vi "SaveTemplate.vi"(11 "Template Name":string) -> ()   [LabVIEW 2019]
uses:
  <userlib>/MicroPython/VIs/ColorText/Code.xctl
panel:
  in  "VISA resource name":refnum<visa-resource-name>
  in  "Open":bool
  in  "Save Button":bool
  in  "Code":string(xcontrol)
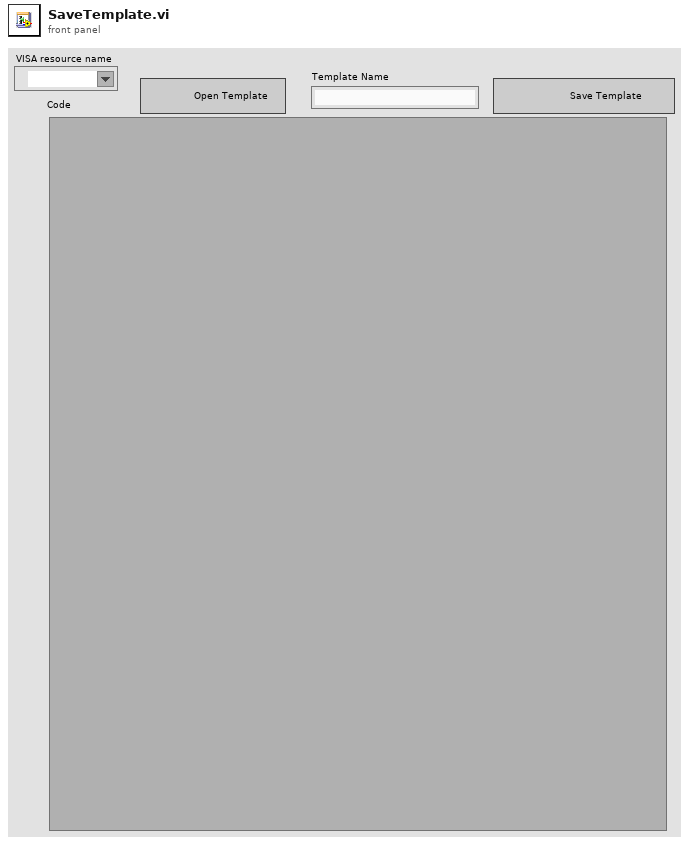
[diagram p1: front panel]
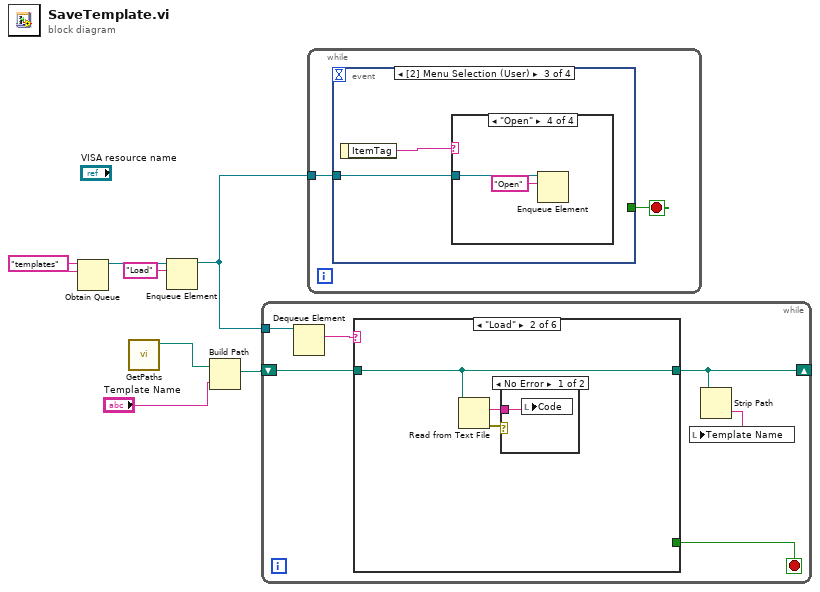
[diagram p0: block diagram]
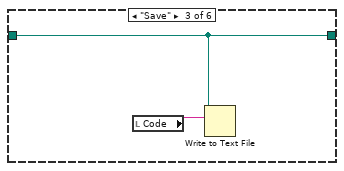
[diagram p4: hidden frame]
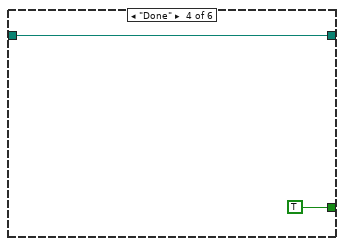
[diagram p5: hidden frame]
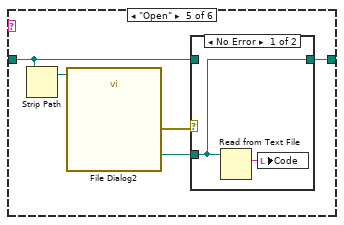
[diagram p6: hidden frame]
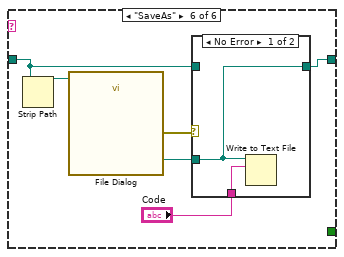
[diagram p8: hidden frame]
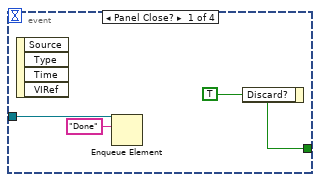
[diagram p10: hidden frame]
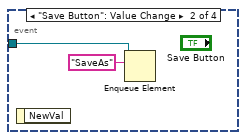
[diagram p11: hidden frame]
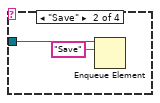
[diagram p13: hidden frame]
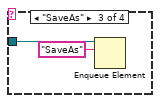
[diagram p14: hidden frame]
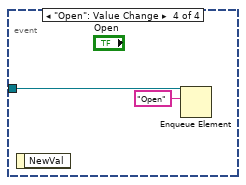
[diagram p15: hidden frame]
diagram:
  w2 = "templates" ("name (unnamed)")
  n1 = Obtain Queue(name (unnamed)=w2, element data type=w2) -> (queue out=w3:refnum<queue>)  [unwired: 3 in, 2 out]
  n2 = call <userlib>:"GetPaths.vi"() -> ("Templates path"=w7:path)  [unwired: 10 in, 1 out]
  n3 = Enqueue Element(queue=w3, element="Load") -> (queue out=w1:refnum<queue>)  [unwired: 2 in, 2 out]
  n4 = Build Path(base path=w7, name or relative path="Template Name") -> (appended path=w5:path)
  n5 = while {
    shift-right: [w9] -> _
    shift-left: w5 -> [w12]
    tunnel: w1 -> [w10]
    stop <- w8 stop-if-true
    n6 = Dequeue Element(queue=w10) -> (element=w13:string)  [unwired: 2 in, 3 out]
    n7 = case shown="\"Load\"" w13 {
      tunnel: [w14 w15 w19 w22 w23 w32] -> w9
      tunnel: w12 -> [w14 w15 w19 w22 w24 w31]
      tunnel: [_ _ _ TRUE _ _] -> w8
      frame Default {
      }
      frame "Load" {
        n8 = Read from Text File(file (use dialog)=w15) -> (text=w16:string, error out=w17:errorcluster)  [unwired: 3 in, 2 out]
        n9 = case shown="No Error" w17 {
          tunnel: w16 -> [w18 _]
          frame No Error {
            n10 = local write "Code"(w18) -> ()
          }
          frame Error {
          }
        }
      }
      frame "Save" {
        n11 = local read "Code"() -> (w20:string)
        n12 = Write to Text File(file (use dialog)=w19, text=w20) -> ()  [unwired: 2 in, 3 out]
      }
      frame "Done" {
      }
      frame "Open" {
        n13 = Strip Path(path=w24) -> (stripped path=w26:path)  [unwired: 1 out]
        n14 = call "File Dialog2"("start path"=w26) -> ("selected path"=w25:path, "error out"=w27:errorcluster)  [unwired: 11 in, 2 out]
        n15 = case shown="No Error" w27 {
          tunnel: w25 -> [w28 _]
          tunnel: [w28 w30] -> w23
          tunnel: w24 -> [_ w30]
          frame No Error {
            n16 = Read from Text File(file (use dialog)=w28) -> (text=w29:string)  [unwired: 3 in, 3 out]
            n17 = local write "Code"(w29) -> ()
          }
          frame Error {
          }
        }
      }
      frame "SaveAs" {
        n18 = Strip Path(path=w31) -> (stripped path=w35:path)  [unwired: 1 out]
        n19 = call "File Dialog"("start path"=w35) -> ("selected path"=w33:path, "error out"=w36:errorcluster)  [unwired: 11 in, 2 out]
        n20 = case shown="No Error" w36 {
          tunnel: w33 -> [w37 _]
          tunnel: "Code" -> [w38 _]
          tunnel: [w37 w39] -> w32
          tunnel: w31 -> [_ w39]
          frame No Error {
            n21 = Write to Text File(file (use dialog)=w37, text=w38) -> ()  [unwired: 2 in, 3 out]
          }
          frame Error {
          }
        }
      }
    }
    n22 = Strip Path(path=w9) -> (name=w11:string)  [unwired: 1 out]
    n23 = local write "Template Name"(w11) -> ()
  }
  n24 = while {
    tunnel: w1 -> [w40]
    stop <- w41 stop-if-true
    n25 = event shown="[2] Menu Selection (User)" {
      selector: _ -> [_ _ _ _]
      dyn-events: _ -> [_ _ _ _]
      timeout: _ -> [_ _ _ _]
      tunnel: [w44 _ _ _] -> w41
      tunnel: w40 -> [w42 w45 w47 w56]
      event Panel Close? {
        w44 = TRUE ("Discard?")
        n26 = event-data() -> ()  [unwired: 1 in, 4 out]
        n27 = Enqueue Element(queue=w42, element="Done") -> ()  [unwired: 2 in, 3 out]
        n28 = event-data("Discard?"=w44) -> ()  [unwired: 1 in, 1 out]
      }
      event "Save Button": Value Change {
        n29 = event-data() -> ()  [unwired: 1 in, 1 out]
        n30 = Enqueue Element(queue=w45, element="SaveAs") -> ()  [unwired: 2 in, 3 out]
      }
      event Menu Selection (User) {
        n31 = event-data() -> ("ItemTag"=w48:string)  [unwired: 1 in]
        n32 = case shown="\"Open\"" w48 {
          tunnel: w47 -> [_ w49 w51 w53]
          frame Default {
          }
          frame "Save" {
            n33 = Enqueue Element(queue=w49, element="Save") -> ()  [unwired: 2 in, 3 out]
          }
          frame "SaveAs" {
            n34 = Enqueue Element(queue=w51, element="SaveAs") -> ()  [unwired: 2 in, 3 out]
          }
          frame "Open" {
            n35 = Enqueue Element(queue=w53, element="Open") -> ()  [unwired: 2 in, 3 out]
          }
        }
      }
      event "Open": Value Change {
        n36 = event-data() -> ()  [unwired: 1 in, 1 out]
        n37 = Enqueue Element(queue=w56, element="Open") -> ()  [unwired: 2 in, 3 out]
      }
    }
  }
